vi "ARES Compass.vi"(8 "Input time of last compass read":dbl, 9 "Compass Com Port":refnum<visa-resource-name>, 10 "Compass In":dbl) -> (3 "Compass Out":dbl, 4 "Output time of last Compass read":dbl)   [LabVIEW 2014]
panel:
  out "Time for Comp?":bool
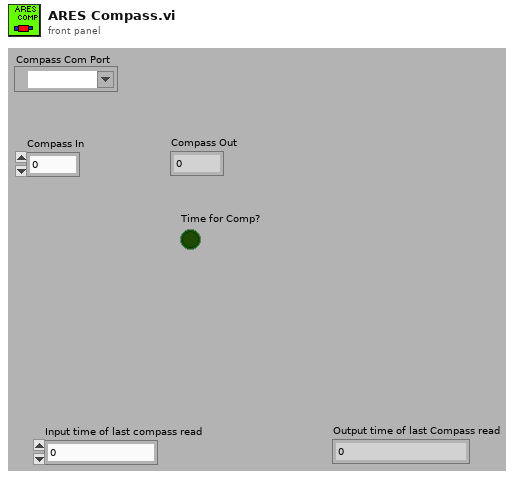
[diagram p1: front panel]
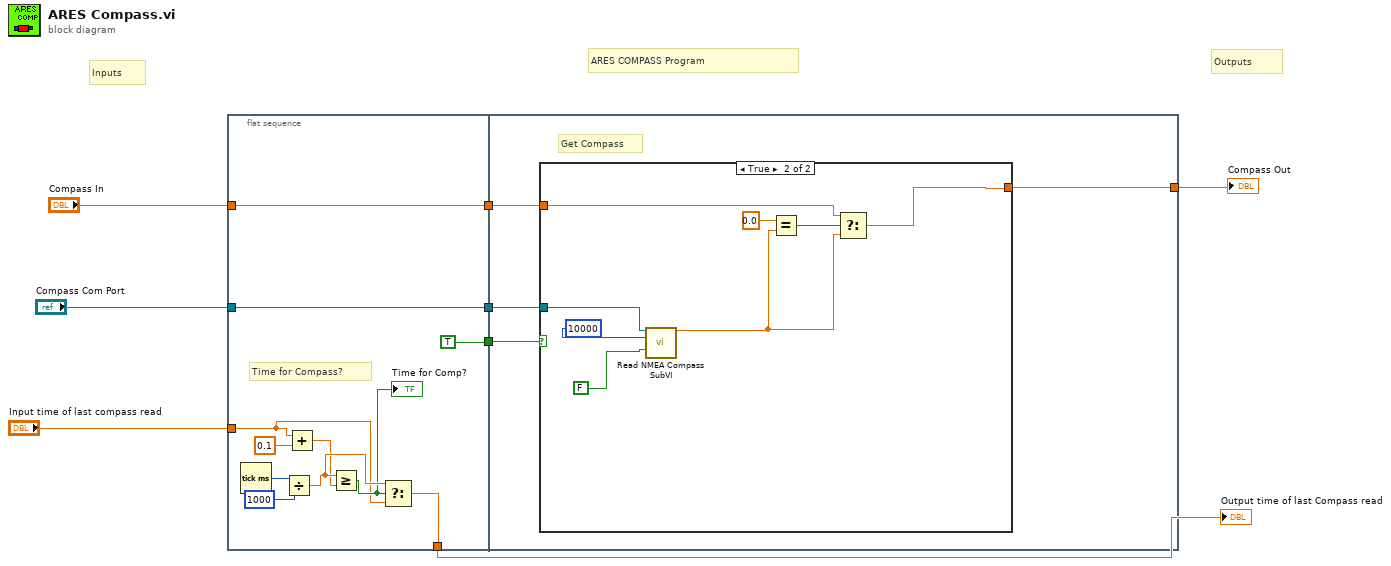
[diagram p0: block diagram]
diagram:
  # "ARES COMPASS Program"
  # "Outputs"
  # "Inputs"
  n1 = flat-sequence {
    tunnel: "Compass Com Port" -> [w19]
    tunnel: [w19] -> w7
    tunnel: [w14] -> w3
    tunnel: [TRUE] -> w6
    tunnel: [w10] -> w5
    tunnel: "Input time of last compass read" -> [w12]
    tunnel: "Compass In" -> [w10]
    tunnel: w7 -> [w23]
    tunnel: w6 -> [w22]
    tunnel: w5 -> [w21]
    tunnel: [w20] -> w1
    frame #0 {
      # "Time for Compass?"
      n2 = Tick Count (ms)() -> (millisecond timer value=w15:u32)
      n3 = Divide(x=w15, y=u32 1000) -> (x/y=w18:dbl)
      n4 = Add(x=w12, y=0.1) -> (x+y=w17:dbl)
      n5 = Greater Or Equal?(x=w18, y=w17) -> (x >= y?=w13:bool)
      "Time for Comp?" <- w13
      n6 = Select(t=w18, s=w13, f=w12) -> (s? t:f=w14:dbl)
    }
    frame #1 {
      # "Get Compass"
      n7 = case shown="True" w22 {
        tunnel: [w24 w28] -> w20
        tunnel: w23 -> [_ w27]
        tunnel: w21 -> [w24 w26]
        frame False {
        }
        frame True {
          n8 = call "Read NMEA Compass SubVI.vi"("VISA resource name"=w27, "timeout (ms)"=u32 10000 ("time out"), "stop"=FALSE) -> ("Heading"=w25:dbl)  [unwired: 10 in, 2 out]
          n9 = Equal?(x=0.0, y=w25) -> (x = y?=w29:bool)
          n10 = Select(t=w26, s=w29, f=w25) -> (s? t:f=w28:dbl)
        }
      }
    }
  }
  "Output time of last Compass read" <- w3
  "Compass Out" <- w1
